vi "Circular Buffer Array LV2012.vi"() -> ()   [LabVIEW 2012]
panel:
  out "Circular Array":i32[](array[numeric])
  in  "Array Size":i32=10
  in  "stop":bool
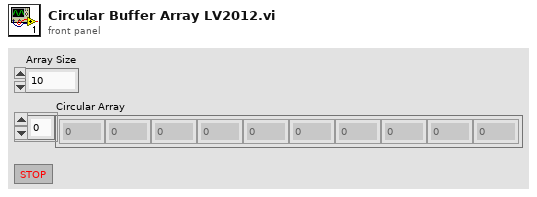
[diagram p1: front panel]
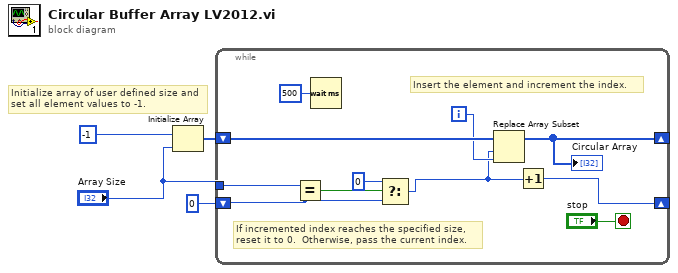
[diagram p0: block diagram]
diagram:
  # "Initialize array of user defined size and set all element values to -1."
  n1 = Initialize Array(-1, "Array Size") -> (w4:i32[])
  n2 = while {
    shift-right: [w14] -> _
    shift-left: 0 -> [w7]
    shift-right: [w12] -> _
    shift-left: w4 -> [w15]
    tunnel: "Array Size" -> [w11]
    i -> [w10]
    stop <- "stop" stop-if-true
    # "If incremented index reaches the specified size, reset it to 0.  Otherwise, pass the current index."
    # "Insert the element and increment the index."
    n3 = Equal?(x=w11, y=w7) -> (x = y?=w8:bool)
    n4 = Wait (ms)(milliseconds to wait=u32 500 ("millisecond multiple")) -> ()  [unwired: 1 out]
    n5 = Select(t=0, s=w8, f=w7) -> (s? t:f=w5:i32)
    n6 = Replace Array Subset "Replace Array Subset"(array=w15, new element=w10, index=w5) -> (w12:i32[])
    "Circular Array" <- w12
    n7 = Increment(x=w5) -> (x+1=w14:i32)
  }
